vi "WallAvoid.vi"() -> ()   [LabVIEW 2012]
panel:
  in  "Lidar Data 0 to 360":dbl[](array[numeric])
  out "WallAvoid Speed":dbl[](array[numeric])
  out "WallAvoid Goodness":dbl[](array[numeric])
  in  "Boat Heading":i32
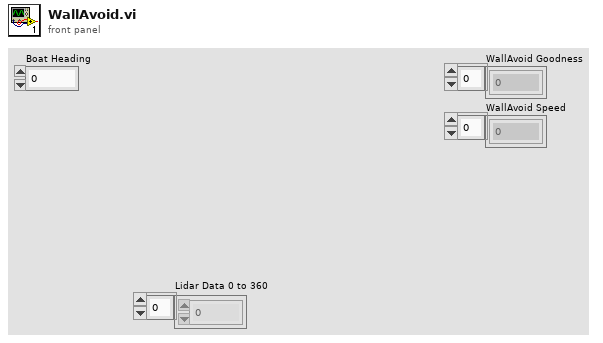
[diagram p1: front panel]
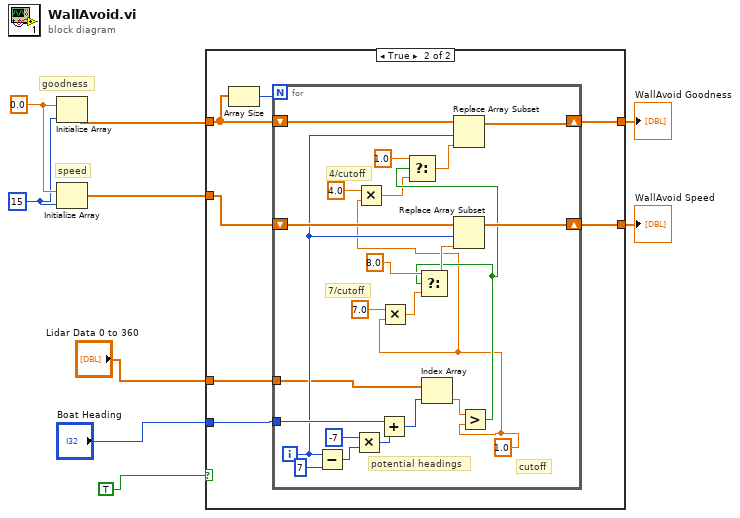
[diagram p0: block diagram]
diagram:
  w8 = 15 ("dimension size")
  w9 = 0.0 ("element")
  # "goodness"
  # "speed"
  n1 = Initialize Array(w9, w8) -> (w5:dbl[])
  n2 = Initialize Array(w9, w8) -> (w4:dbl[])
  n3 = case shown="True" TRUE {
    tunnel: "Boat Heading" -> [_ w18]
    tunnel: w5 -> [w11 w16]
    tunnel: w4 -> [w10 w15]
    tunnel: [w11 w14] -> w3
    tunnel: [w10 w13] -> w2
    tunnel: "Lidar Data 0 to 360" -> [_ w12]
    frame False {
    }
    frame True {
      n4 = Array Size(array=w16) -> (size(s)=w17:i32)
      n5 = for {
        N: w17 -> [_]
        tunnel: w18 -> [w37]
        shift-right: [w34] -> w14
        shift-left: w16 -> [w36]
        shift-right: [w33] -> w13
        shift-left: w15 -> [w35]
        tunnel: w12 -> [w31]
        i -> [w32]
        w20 = 1.0 ("y")
        # "4/cutoff"
        # "7/cutoff"
        # "cutoff"
        # "potential headings"
        n6 = Subtract(x=w32, y=7) -> (x-y=w40:i32)
        n7 = Multiply(x=-7, y=w40) -> (x*y=w38:i32)
        n8 = Multiply(x=4.0, y=w20) -> (x*y=w19:dbl)
        n9 = Add(x=w37, y=w38) -> (x+y=w30:i32)
        n10 = Multiply(x=7.0, y=w20) -> (x*y=w27:dbl)
        n11 = Index Array(array=w31, index=w30) -> (element=w29:dbl)
        n12 = Greater?(x=w29, y=w20) -> (0:w22:bool)
        n13 = Select(t=1.0, s=w22, f=w19) -> (s? t:f=w24:dbl)
        n14 = Select(t=8.0, s=w22, f=w27) -> (s? t:f=w25:dbl)
        n15 = Replace Array Subset(array=w36, new element=w24, index=w32) -> (w34:dbl[])
        n16 = Replace Array Subset(array=w35, new element=w25, index=w32) -> (w33:dbl[])
      }
    }
  }
  "WallAvoid Goodness" <- w3
  "WallAvoid Speed" <- w2
